vi "thermistor_reduced_R.vi"(8 "ready for output (T)":bool=TRUE, 9 "input valid":bool=TRUE, 10 "V":fxp<+/-,24,5>, 11 "1/R_inf":fxp<+,32,7>) -> (0 "ready for input":bool, 1 "output valid":bool, 2 "R^~":fxp<+/-,64,32>)   [LabVIEW 2018]
uses:
  <vilib>/rvi/FXPMathLib/FxpDiv/subVIs/nifxpmath_Div_SimConfig.ctl
  <vilib>/rvi/FXPMathLib/FxpDiv/simVIs/DllFxpDivTemp_sub.vi
  <vilib>/rvi/FXPMathLib/FxpSub/XNode/nifxpmath_Sub.xnode
  <vilib>/rvi/FXPMathLib/FxpMul/XNode/nifxpmath_Multiplier.xnode
  <vilib>/rvi/FXPMathLib/FxpDiv/XNode/nifxpmath_Div.xnode
  <vilib>/rvi/FXPMathLib/sim/FxpSim.dll
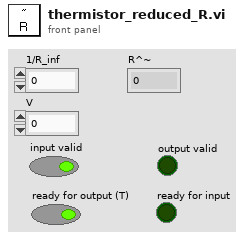
[diagram p1: front panel]
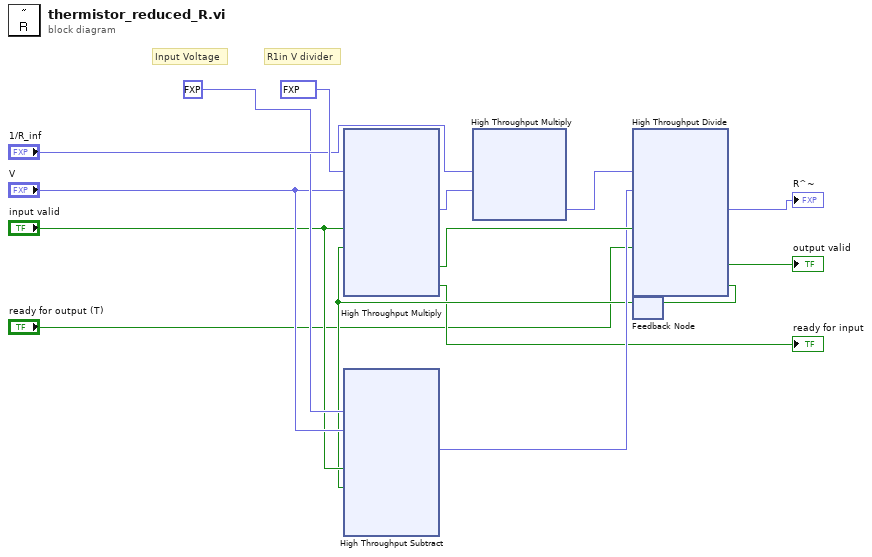
[diagram p0: block diagram]
diagram:
  # "Input Voltage"
  # "R1in V divider"
  n1 = feedback #1() -> (w5:bool)  [unwired: 1 in]
  n2 = xnode "High Throughput Multiply"("x"=fxp<+,10,14> 10000.0 ("y"), "y"="V", "input valid"="input valid", "ready for output (T)"=w5) -> ("x*y"=w14:fxp<+/-,34,19>, "output valid"=w9:bool, "ready for input"=→"ready for input":bool)
  n3 = xnode "High Throughput Subtract"("x"=fxp<+,3,5> 24.0, "y"="V", "input valid"="input valid", "ready for output (T)"=w5) -> ("x-y"=w8:fxp<+/-,23,7>)  [unwired: 2 out]
  n4 = xnode "High Throughput Multiply"("x"="1/R_inf", "y"=w14) -> ("x*y"=w7:fxp<+/-,64,26>)
  n5 = xnode "High Throughput Divide"("x"=w7, "y"=w8, "input valid"=w9, "ready for output (T)"="ready for output (T)") -> ("x/y"=→"R^~":fxp<+/-,64,32>, "output valid"=→"output valid":bool, "ready for input"=w6:bool)
  n6 = feedback-in #1(w6) -> ()
